vi "Write Cylinder.vi"(10 "ActuatorCylinder":refnum<class "IActuatorCylinder.lvclass">, 11 "PressureServoActuator in":refnum<class "PressureServoActuatorClosed.lvclass">) -> (3 "PressureServoActuator out":refnum<class "PressureServoActuatorClosed.lvclass">)   [LabVIEW 2015, in "PressureServoActuatorClosed.lvclass"]
uses:
  PressureServoActuatorClosed.lvclass
  ActuatorCylinder/IActuatorCylinder/IActuatorCylinder.lvclass
  PressureServoActuatorClosed.lvclass/PressureServoActuatorClosed.ctl
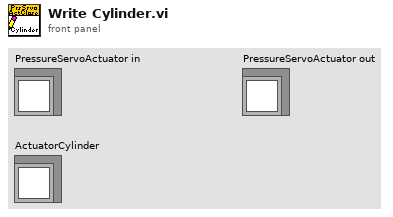
[diagram p1: front panel]
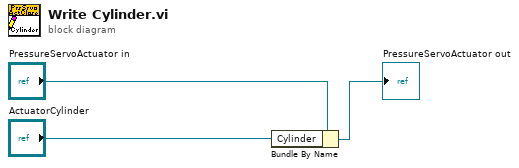
[diagram p0: block diagram]
diagram:
  n1 = Bundle By Name(cluster="PressureServoActuator in", "Cylinder"="ActuatorCylinder") -> (→"PressureServoActuator out":refnum<class "PressureServoActuatorClosed.lvclass">)
